vi "Planecontrols.vi"() -> ()   [LabVIEW 2015]
uses:
  <vilib>/DAQmx/read.llb/DAQmx Read (Analog Wfm 1Chan NSamp).vi
  <vilib>/DAQmx/create/channels.llb/DAQmx Create Channel (AI-Voltage-Basic).vi
  <vilib>/DAQmx/configure/timing.llb/DAQmx Timing (Sample Clock).vi
  global.vi
  <vilib>/DAQmx/miscellaneous.llb/DAQmx Fill In Error Info.vi
panel:
  out "Altitude":dbl
  out "Iterations":i32
  out "Light Sensor":dbl
  out "Roll":dbl
  out "Airspeed":dbl
  out "Boolean":bool
  in  "Wing Tips":bool
  out "Previous Speed":dbl
  out "?":bool
  out "?":bool
  out "?":bool
  out "?":bool
  in  "Current Speed":dbl(slide) scale=0.0..400.0
  in  "Roll Slider":dbl(slide) scale=-90.0..90.0
  in  "Fan":bool
  in  "Breaks":bool
  in  "Right Indicator":bool
  in  "Left Indicator":bool
  out "Waveform Graph":waveform(dbl)(graph)
  in  "?":bool
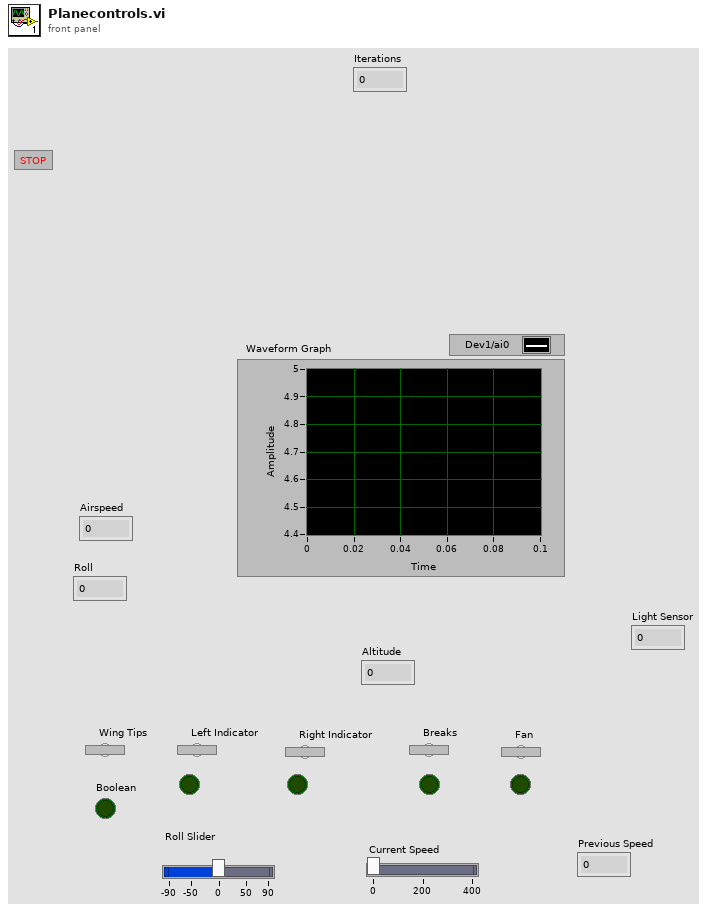
[diagram p1: front panel]
types:
  T1 = cluster{"Airspeed":dbl, "Altitude":dbl, "Vertical Speed":dbl, "Pitch":dbl, "Roll":dbl, "Heading":dbl, "Turn Indicator":dbl, "Latitude":dbl, "Longitude":dbl}
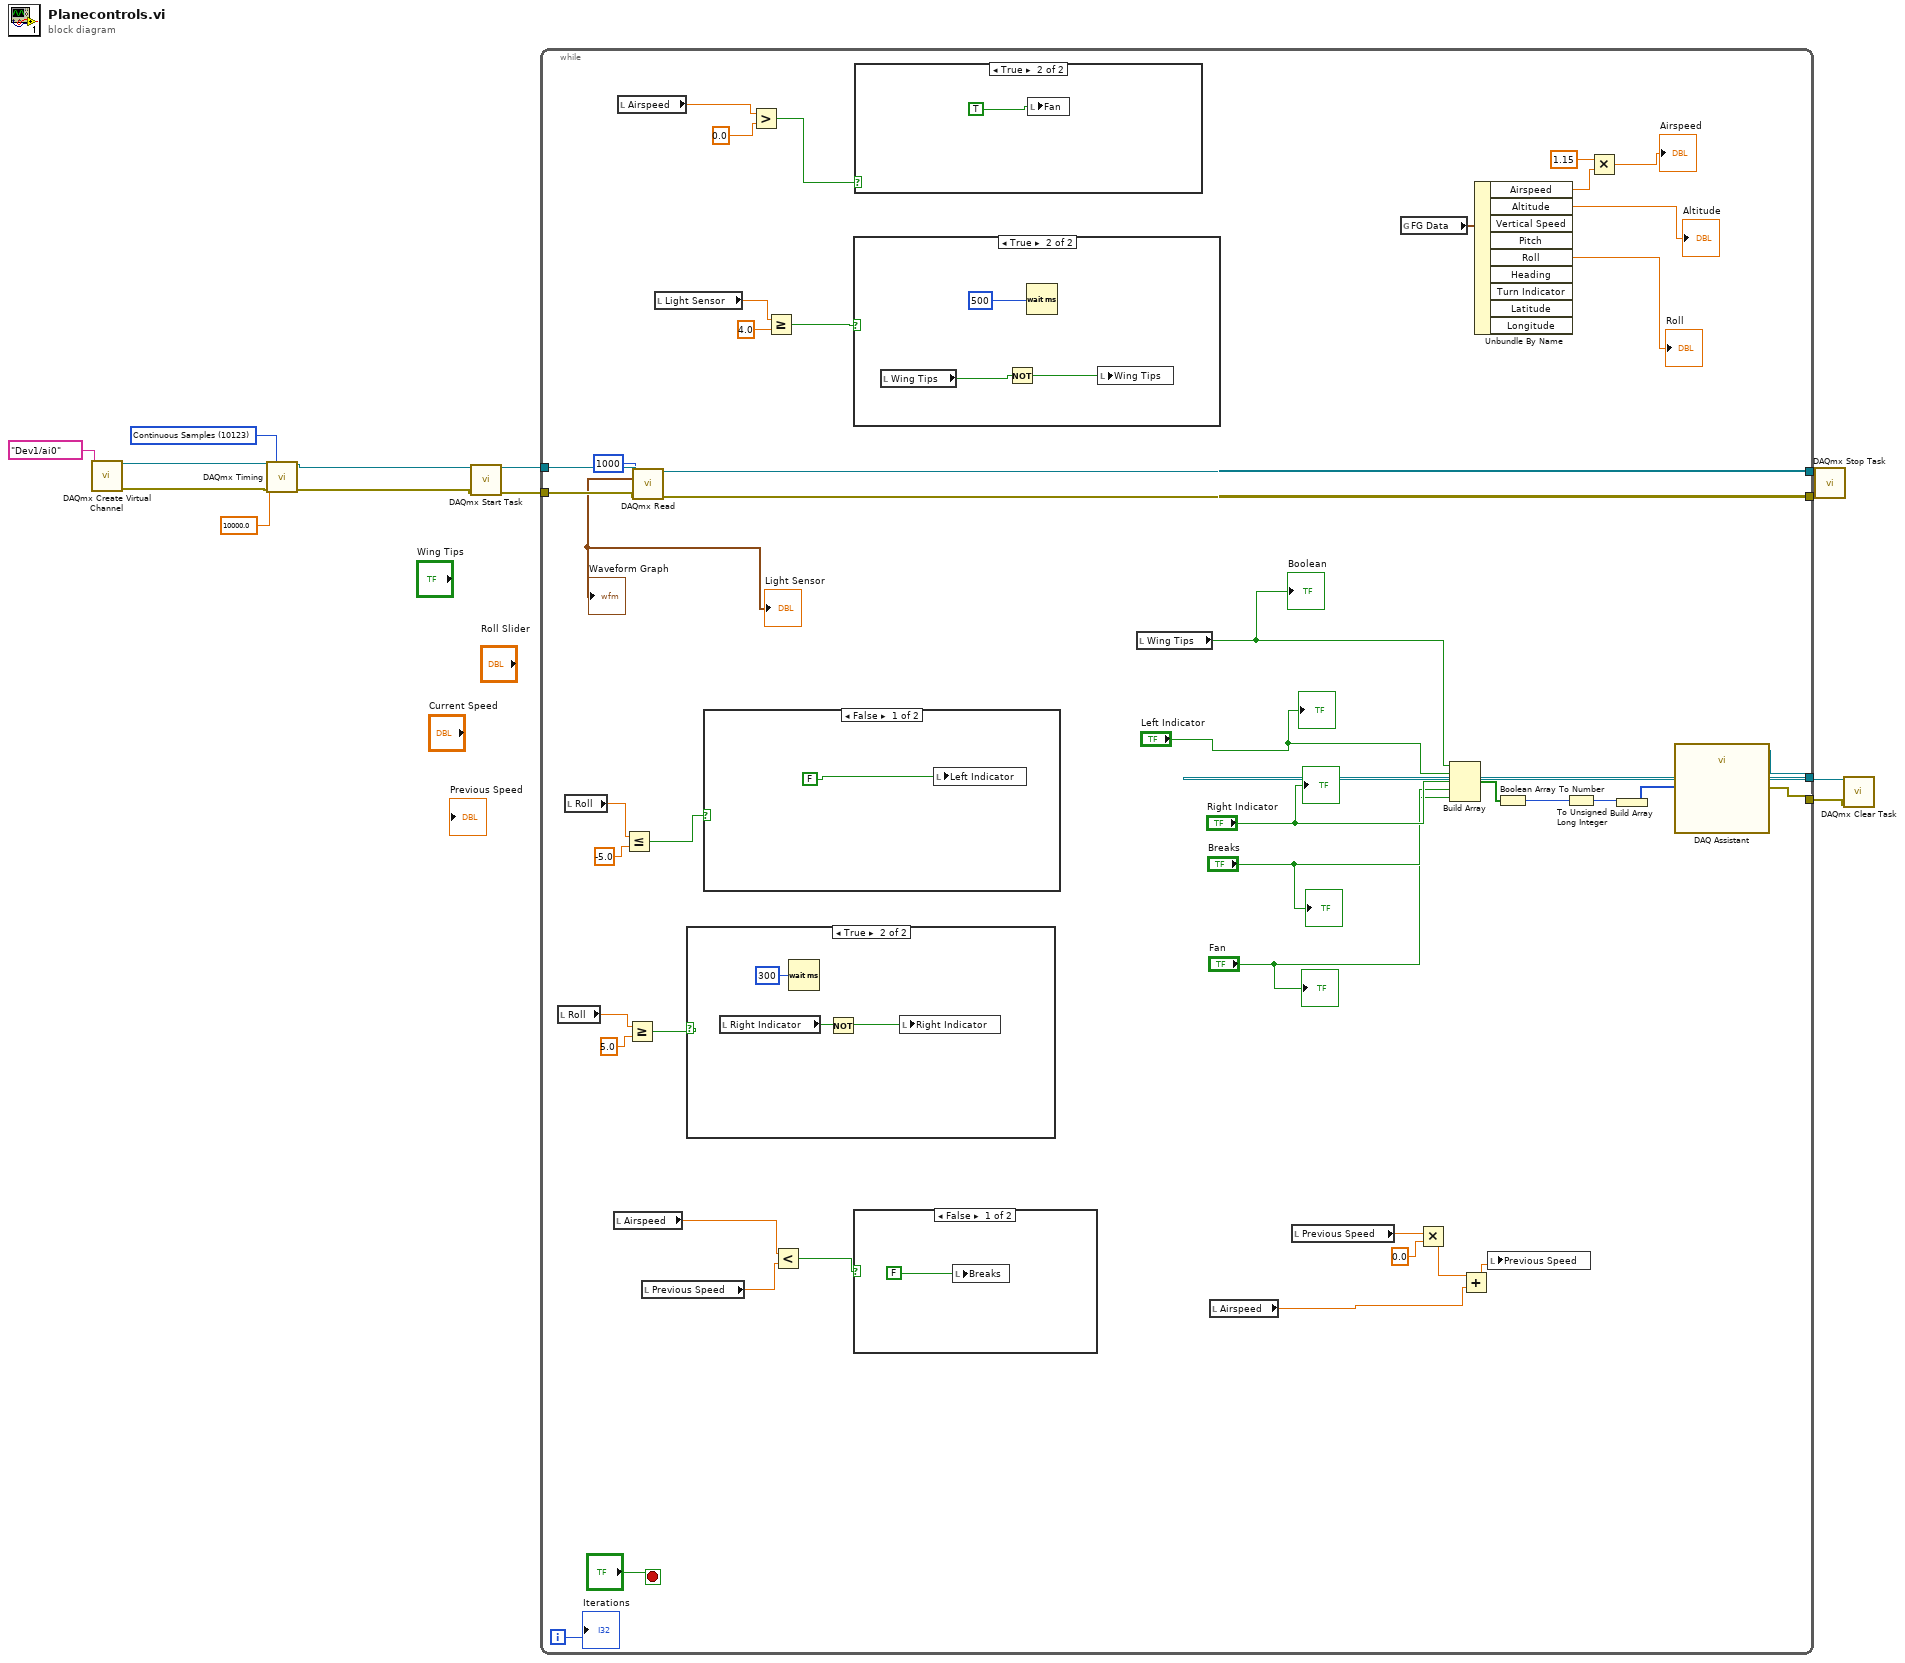
[diagram p0: block diagram]
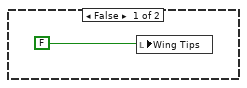
[diagram p2: hidden frame]
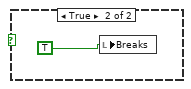
[diagram p3: hidden frame]
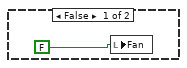
[diagram p4: hidden frame]
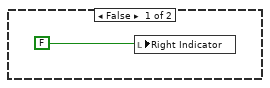
[diagram p5: hidden frame]
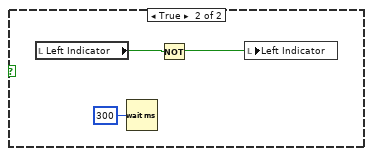
[diagram p6: hidden frame]
diagram:
  w11 = 10123 items=["Finite Samples"=10178, "Continuous Samples"=10123, "Hardware Timed Single Point"=12522] ("sample mode")
  n1 = call-poly <vilib>:"DAQmx Create Virtual Channel.vi"("physical channels"=tag "Dev1/ai0") -> ("task out"=w12:refnum<k21>, "error out"=w9:errorcluster)  [unwired: 13 in]
  n2 = call-poly <vilib>:"DAQmx Timing.vi"("task/channels in"=w12, "sample mode"=w11, "rate"=10000.0, "error in"=w9) -> ("task out"=w5:refnum<k21>, "error out"=w8:errorcluster)  [unwired: 10 in]
  n3 = call <vilib>:"DAQmx Start Task.vi"("task/channels in"=w5, "error in"=w8) -> ("task out"=w6:refnum<k21>, "error out"=w7:errorcluster)  [unwired: 12 in]
  n4 = while {
    tunnel: w7 -> [w58]
    tunnel: w6 -> [w57]
    tunnel: [w55] -> w4
    tunnel: [w54] -> w3
    tunnel: [w51] -> w2
    tunnel: [w50] -> w1
    i -> [w16]
    stop <- "?" stop-if-true
    n5 = local read "Roll"() -> (w20:dbl)
    n6 = local read "Roll"() -> (w21:dbl)
    n7 = local read "Airspeed"() -> (w27:dbl)
    n8 = local read "Airspeed"() -> (w25:dbl)
    n9 = Less Or Equal?(x=w21, y=-5.0) -> (x <= y?=w45:bool)
    n10 = Greater Or Equal?(x=w20, y=5.0) -> (x >= y?=w43:bool)
    n11 = call-poly <vilib>:"DAQmx Read.vi"("task/channels in"=w57, "number of samples per channel"=1000, "error in"=w58) -> ("task out"=w54:refnum<k21>, "data"=→"Waveform Graph" →"Light Sensor":waveform(dbl), "error out"=w55:errorcluster)  [unwired: 10 in]
    n12 = local read "Previous Speed"() -> (w35:dbl)
    n13 = local read "Light Sensor"() -> (w18:dbl)
    n14 = case shown="True" w43 {
      frame False {
        n15 = local write "Right Indicator"(FALSE) -> ()
      }
      frame True {
        n16 = local read "Right Indicator"() -> (w69:bool)
        n17 = Wait (ms)(milliseconds to wait=u32 300) -> ()  [unwired: 1 out]
        n18 = Not(x=w69) -> (.not. x?=w70:bool)
        n19 = local write "Right Indicator"(w70) -> ()
      }
    }
    n20 = case shown="False" w45 {
      frame False {
        n21 = local write "Left Indicator"(FALSE) -> ()
      }
      frame True {
        n22 = local read "Left Indicator"() -> (w73:bool)
        n23 = Wait (ms)(milliseconds to wait=u32 300) -> ()  [unwired: 1 out]
        n24 = Not(x=w73) -> (.not. x?=w74:bool)
        n25 = local write "Left Indicator"(w74) -> ()
      }
    }
    n26 = Greater?(x=w25, y=0.0 ("x")) -> (0:w38:bool)
    n27 = Greater Or Equal?(x=w18, y=4.0) -> (x >= y?=w14:bool)
    n28 = Less?(x=w27, y=w35) -> (x < y?=w34:bool)
    n29 = case shown="True" w14 {
      frame False {
        n30 = local write "Wing Tips"(FALSE) -> ()
      }
      frame True {
        n31 = local read "Wing Tips"() -> (w61:bool)
        n32 = Not(x=w61) -> (.not. x?=w62:bool)
        n33 = Wait (ms)(milliseconds to wait=u32 500 ("millisecond timer value")) -> ()  [unwired: 1 out]
        n34 = local write "Wing Tips"(w62) -> ()
      }
    }
    n35 = case shown="False" w34 {
      frame False {
        n36 = local write "Breaks"(FALSE) -> ()
      }
      frame True {
        n37 = local write "Breaks"(TRUE) -> ()
      }
    }
    n38 = case shown="True" w38 {
      frame False {
        n39 = local write "Fan"(FALSE) -> ()
      }
      frame True {
        n40 = local write "Fan"(TRUE) -> ()
      }
    }
    n41 = local read "Wing Tips"() -> (w36:bool)
    "Boolean" <- w36
    n42 = local read "Airspeed"() -> (w26:dbl)
    n43 = local read "Previous Speed"() -> (w31:dbl)
    n44 = global read "Global.vi" "FG Data"() -> (w29:T1)
    n45 = Multiply(x=w31, y=0.0) -> (x*y=w32:dbl)
    n46 = Build Array(w36, "Left Indicator", "Right Indicator", "Breaks", "Fan") -> (w49:bool[])
    n47 = Add(x=w32, y=w26) -> (x+y=w33:dbl)
    n48 = Unbundle By Name(w29) -> ("Airspeed"=w24:dbl, "Altitude"=→"Altitude":dbl, "Roll"=→"Roll":dbl)  [unwired: 6 out]
    n49 = local write "Previous Speed"(w33) -> ()
    n50 = Boolean Array To Number(Boolean array=w49) -> (number=w52:u32)
    n51 = To Unsigned Long Integer(number=w52) -> (unsigned 32bit integer=w48:u32)
    n52 = Multiply(x=1.15, y=w24) -> (x*y=→"Airspeed":dbl)
    n53 = Build Array(w48) -> (w47:u32[])
    n54 = call "DAQ Assistant"("data"=w47) -> ("task out"=w51:refnum<k21>, "error out"=w50:errorcluster)  [unwired: 17 in]
    "?" <- "Left Indicator"
    "?" <- "Right Indicator"
    "?" <- "Breaks"
    "?" <- "Fan"
    "Iterations" <- w16
  }
  n55 = call <vilib>:"DAQmx Stop Task.vi"("task/channels in"=w3, "error in"=w4) -> ()  [unwired: 12 in, 2 out]
  n56 = call <vilib>:"DAQmx Clear Task.vi"("task in"=w2, "error in"=w1) -> ()  [unwired: 13 in, 1 out]
